vi "TrajectoryCreateExecuteAbsolutePointInFront.vi"(8 "Init":bool, 11 "End Pose ENG":T1={"TRANSLATION"={"X"=0.0, "Y"=0.0}, "ROTATION"={"VALUE"=0.0, "COS"=1.0, "SIN"=0.0}} {"ROTATION"."SIN" format="%13.4f"; "ROTATION"."COS" format="%13.4f"; "ROTATION"."VALUE" format="%13.4f"; "TRANSLATION"."Y" format="%14.3f"; "TRANSLATION"."X" format="%14.3f"}) -> (0 "AtReference":bool, 3 "Chassis Velocity Target":T4 {"vOmega" format="%10.3f"; "vY" format="%10.3f"; "vX" format="%10.3f"})   [LabVIEW 2023]
uses:
  <vilib>/Rock Robotics/WPI/ThirdParty/JAS_Junk/TrajLib/TypeDef/CHASSIS_SPEEDS.ctl
  <vilib>/Rock Robotics/WPI/ThirdParty/JAS_Junk/TrajLib/TypeDef/POSE2D.ctl
  <vilib>/Rock Robotics/WPI/ThirdParty/JAS_Junk/TrajLib/TypeDef/TRANSLATION2D.ctl
  <vilib>/Rock Robotics/WPI/ThirdParty/JAS_Junk/TrajLib/TypeDef/ROTATION2D.ctl
  <vilib>/Rock Robotics/WPI/ThirdParty/JAS_Junk/TrajLib/VI/Util_GetTime_U32.vi
  <vilib>/Rock Robotics/WPI/ThirdParty/JAS_Junk/TrajLib/HolDrvCtrl_New.vi
  <vilib>/Rock Robotics/WPI/ThirdParty/JAS_Junk/TrajLib/HolDrvCtrl_PackPID.vi
  <vilib>/Rock Robotics/WPI/ThirdParty/JAS_Junk/TrajLib/HolDrvCtrl_SetTolerance.vi
  <vilib>/Rock Robotics/WPI/ThirdParty/JAS_Junk/TrajLib/HolDrvCtrl_SetEnabled.vi
  <vilib>/Rock Robotics/WPI/ThirdParty/JAS_Junk/TrajLib/HolDrvCtrl_Calculate_Trajectory.vi
  <vilib>/Rock Robotics/WPI/ThirdParty/JAS_Junk/TrajLib/HolDrvCtrl_AtReference.vi
  <vilib>/Rock Robotics/WPI/ThirdParty/JAS_Junk/TrajLib/ProfiledPIDController_NewPeriod.vi
  <vilib>/Rock Robotics/WPI/ThirdParty/JAS_Junk/TrajLib/ProfiledPIDController_SetIntegratorRange.vi
  <vilib>/Rock Robotics/WPI/ThirdParty/JAS_Junk/TrajLib/ProfiledPIDController_DisableContInput.vi
  <vilib>/Rock Robotics/WPI/ThirdParty/JAS_Junk/TrajLib/ProfiledPIDController_EnableContInput.vi
  <vilib>/Rock Robotics/WPI/ThirdParty/JAS_Junk/TrajLib/TrapProfConstraint_New.vi
  <vilib>/Rock Robotics/WPI/ThirdParty/JAS_Junk/TrajLib/Rotation2d_CreateAngle.vi
  <vilib>/Rock Robotics/WPI/ThirdParty/JAS_Junk/TrajLib/Translation2d_GetXY.vi
  <vilib>/Rock Robotics/WPI/ThirdParty/JAS_Junk/TrajLib/Rotation2d_CreateXY.vi
  <vilib>/Rock Robotics/WPI/ThirdParty/JAS_Junk/TrajLib/Rotation2d_GetRadians.vi
  <vilib>/Rock Robotics/WPI/ThirdParty/JAS_Junk/TrajLib/Conv_Deg_Radians.vi
  <vilib>/Rock Robotics/WPI/ThirdParty/JAS_Junk/TrajLib/PIDController_NewPeriod.vi
  <vilib>/Rock Robotics/WPI/ThirdParty/JAS_Junk/TrajLib/PIDController_SetIntegratorRange.vi
  <vilib>/Rock Robotics/WPI/ThirdParty/JAS_Junk/TrajLib/PIDController_Reset.vi
  <vilib>/Rock Robotics/WPI/ThirdParty/JAS_Junk/TrajLib/HolDrvCtrl_Calculate.vi
  <vilib>/Rock Robotics/WPI/ThirdParty/JAS_Junk/TrajLib/TrapProfState_New.vi
  <vilib>/Rock Robotics/SystemInterfaces/NetworkCommunication/NetComm_UsageReport_report.vi
  <vilib>/Rock Robotics/WPI/ThirdParty/JAS_Junk/TrajLib/PIDController_DisableContinousInput.vi
  <vilib>/Rock Robotics/WPI/ThirdParty/JAS_Junk/TrajLib/PIDController_EnableContinousInput.vi
  <vilib>/Rock Robotics/WPI/ThirdParty/JAS_Junk/TrajLib/Util_CalcDist.vi
  <vilib>/Rock Robotics/WPI/ThirdParty/JAS_Junk/TrajLib/Rotation2d_GetAngleCosSin.vi
  <vilib>/Rock Robotics/WPI/ThirdParty/JAS_Junk/TrajLib/Pose2d_RelativeTo.vi
  <vilib>/Rock Robotics/WPI/ThirdParty/JAS_Junk/TrajLib/Pose2d_getRotation.vi
  <vilib>/Rock Robotics/WPI/ThirdParty/JAS_Junk/TrajLib/Rotation2d_Minus.vi
  <vilib>/Rock Robotics/WPI/ThirdParty/JAS_Junk/TrajLib/ProfiledPIDController_Calculate_Meas_Goal.vi
  <vilib>/Rock Robotics/WPI/ThirdParty/JAS_Junk/TrajLib/PIDController_Calculate_SP_PV.vi
  <vilib>/Rock Robotics/WPI/ThirdParty/JAS_Junk/TrajLib/ProfiledPIDController_Reset_PosOnly.vi
  <vilib>/Rock Robotics/WPI/ThirdParty/JAS_Junk/TrajLib/ChassisSpeeds_FromFieldRelativeSpeeds.vi
  <vilib>/Rock Robotics/WPI/ThirdParty/JAS_Junk/TrajLib/Transform2d_Create_PosePose.vi
  <vilib>/Rock Robotics/WPI/ThirdParty/JAS_Junk/TrajLib/Pose2d_New_TRRO.vi
  <vilib>/Rock Robotics/WPI/ThirdParty/JAS_Junk/TrajLib/Rotation2d_UnaryMinus.vi
  <vilib>/Rock Robotics/WPI/ThirdParty/JAS_Junk/TrajLib/Rotation2d_RotateBy.vi
  <vilib>/Rock Robotics/WPI/ThirdParty/JAS_Junk/TrajLib/ProfiledPIDController_SetGoal_PosOnly.vi
  <vilib>/Rock Robotics/WPI/ThirdParty/JAS_Junk/TrajLib/ProfiledPIDController_Calculate_Meas.vi
  <vilib>/Rock Robotics/WPI/ThirdParty/JAS_Junk/TrajLib/PIDController_SetSetpoint.vi
  <vilib>/Rock Robotics/WPI/ThirdParty/JAS_Junk/TrajLib/PIDController_Calculate_PV.vi
  <vilib>/Rock Robotics/WPI/ThirdParty/JAS_Junk/TrajLib/ProfiledPIDController_Reset.vi
  <vilib>/Rock Robotics/WPI/ThirdParty/JAS_Junk/TrajLib/Rotation2d_GetCos.vi
  <vilib>/Rock Robotics/WPI/ThirdParty/JAS_Junk/TrajLib/Rotation2d_GetSin.vi
  <vilib>/Rock Robotics/WPI/ThirdParty/JAS_Junk/TrajLib/Translation2d_RotateBy.vi
  <vilib>/Rock Robotics/WPI/ThirdParty/JAS_Junk/TrajLib/ProfiledPIDController_SetGoal.vi
  <vilib>/Rock Robotics/WPI/ThirdParty/JAS_Junk/TrajLib/TrapProfile_New.vi
  <vilib>/Rock Robotics/WPI/ThirdParty/JAS_Junk/TrajLib/ProfiledPIDController_GetPeriod.vi
  <vilib>/Rock Robotics/WPI/ThirdParty/JAS_Junk/TrajLib/TrapProfile_Calculate.vi
  <vilib>/Rock Robotics/WPI/ThirdParty/JAS_Junk/TrajLib/ControllerUtil_GetModulusError.vi
  <vilib>/Rock Robotics/WPI/ThirdParty/JAS_Junk/TrajLib/TrapProfile_ShouldFlipAcceleration.vi
  <vilib>/Rock Robotics/WPI/ThirdParty/JAS_Junk/TrajLib/TrapProfile_Direct.vi
  <vilib>/Rock Robotics/WPI/ThirdParty/JAS_Junk/TrajLib/PIDController_GetPeriod.vi
  Vision/VisionGlobal.vi
  TrajectoryGlobals.vi
  <vilib>/Rock Robotics/SystemInterfaces/Utilities/FPGA_UtilitiesRead LocalTime.vi
  <vilib>/Rock Robotics/WPI/ThirdParty/JAS_Junk/TrajLib/VI/Util_GetTime_U64.vi
  <vilib>/Rock Robotics/WPI/ThirdParty/JAS_Junk/TrajLib/Globals/Util_LibraryGlobals.vi
  <vilib>/Rock Robotics/WPI/ThirdParty/JAS_Junk/TrajLib/Trajectory_Library.lvlib
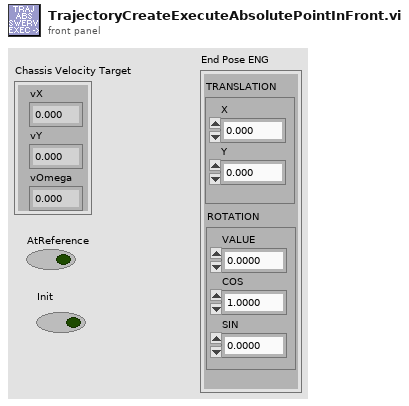
[diagram p1: front panel]
types:
  T1 = typedef "Trajectory_Library.lvlib/POSE2D.ctl" = cluster{"TRANSLATION":T2, "ROTATION":T3}
  T2 = typedef "Trajectory_Library.lvlib/TRANSLATION2D.ctl" = cluster{"X":dbl, "Y":dbl}
  T3 = typedef "Trajectory_Library.lvlib/ROTATION2D.ctl" = cluster{"VALUE":dbl, "COS":dbl, "SIN":dbl}
  T4 = typedef "Trajectory_Library.lvlib/CHASSIS_SPEEDS.ctl" = cluster{"vX":dbl, "vY":dbl, "vOmega":dbl}
  T5 = typedef "Trajectory_Library.lvlib/SWERVE_DRIVE_KINEMATICS.ctl" = cluster{"NumModules":i32, "InverseKinematics":T6, "ForwardKinematics":T6, "Modules":T2[], "PrevCoR":T2, "SavedModuleStates":T7[]}
  T6 = typedef "NI_Matrix.lvlib/RealMatrix.ctl" = dbl[][]
  T7 = typedef "Trajectory_Library.lvlib/SWERVE_DRIVE_MODULE_STATE.ctl" = cluster{"Speed":dbl, "Angle":T3}
  T8 = typedef "Trajectory_Library.lvlib/TRAJECTORY.ctl" = cluster{"TotalTImeSecs":dbl, "States":T9[]}
  T9 = typedef "Trajectory_Library.lvlib/TRAJ_STATE.ctl" = cluster{"TimeSeconds":dbl, "Velocity":dbl, "Acceleration":dbl, "POSE":T1, "Curvature":dbl}
  T10 = typedef "Trajectory_Library.lvlib/PID_TUNING.ctl" = cluster{"Kp":dbl, "Ki":dbl, "Kd":dbl, "MaximumIntegral":dbl, "MinimumIntegral":dbl, "IntegralZone":dbl}
  T11 = typedef "Trajectory_Library.lvlib/PROFILED_PID_CONTROLLER.ctl" = cluster{"Controller":T12, "Goal":T13, "Setpoint":T13, "Constraint":T14}
  T12 = typedef "Trajectory_Library.lvlib/PID_CONTROLLER.ctl" = cluster{"Kp":dbl, "Ki":dbl, "Kd":dbl, "Period":dbl, "Max_Integral":dbl, "Min_Integral":dbl, "Max_Input":dbl, "Min_Input":dbl, "Continuous":bool, "PositionError":dbl, "VelocityError":dbl, "PrevError":dbl, "Total_Integral":dbl, "PositionTolerance":dbl, "VelocityTolerance":dbl, "SetPoint":dbl, "Kf":dbl, "Prev_Deriv":dbl, "Prev_Deriv 2":dbl, "DerivativeFilter":bool, "Min_Output":dbl, "Max_Output":dbl, "Prev_F_P":dbl, "Prev_F_P_2":dbl, "AntiWindupActive":bool, "Measurement":dbl, "IntegralZone":dbl}
  T13 = typedef "Trajectory_Library.lvlib/TRAPEZOID_PROFILE_STATE.ctl" = cluster{"Position":dbl, "Velocity":dbl}
  T14 = typedef "Trajectory_Library.lvlib/TRAPEZOID_PROFILE_CONSTRAINT.ctl" = cluster{"MaxVelocity":dbl, "MaxAcceleration":dbl}
  T15 = typedef "Trajectory_Library.lvlib/HOLONOMIC_PACK_TUNING.ctl" = cluster{"X PID Tuning":T10, "Y PID Tuning":T10, "thetaProfiledPID_CTRL":T11}
  T16 = typedef "Trajectory_Library.lvlib/HOLONOMIC_DRV_CTRL.ctl" = cluster{"poseTolerance":T1, "poseError":T1, "Enabled":bool, "PID_xCtrl":T12, "PID_yCtrl":T12, "PROF_PID_thetaCtrl":T11, "RotationError":T3, "FirstRun":bool}
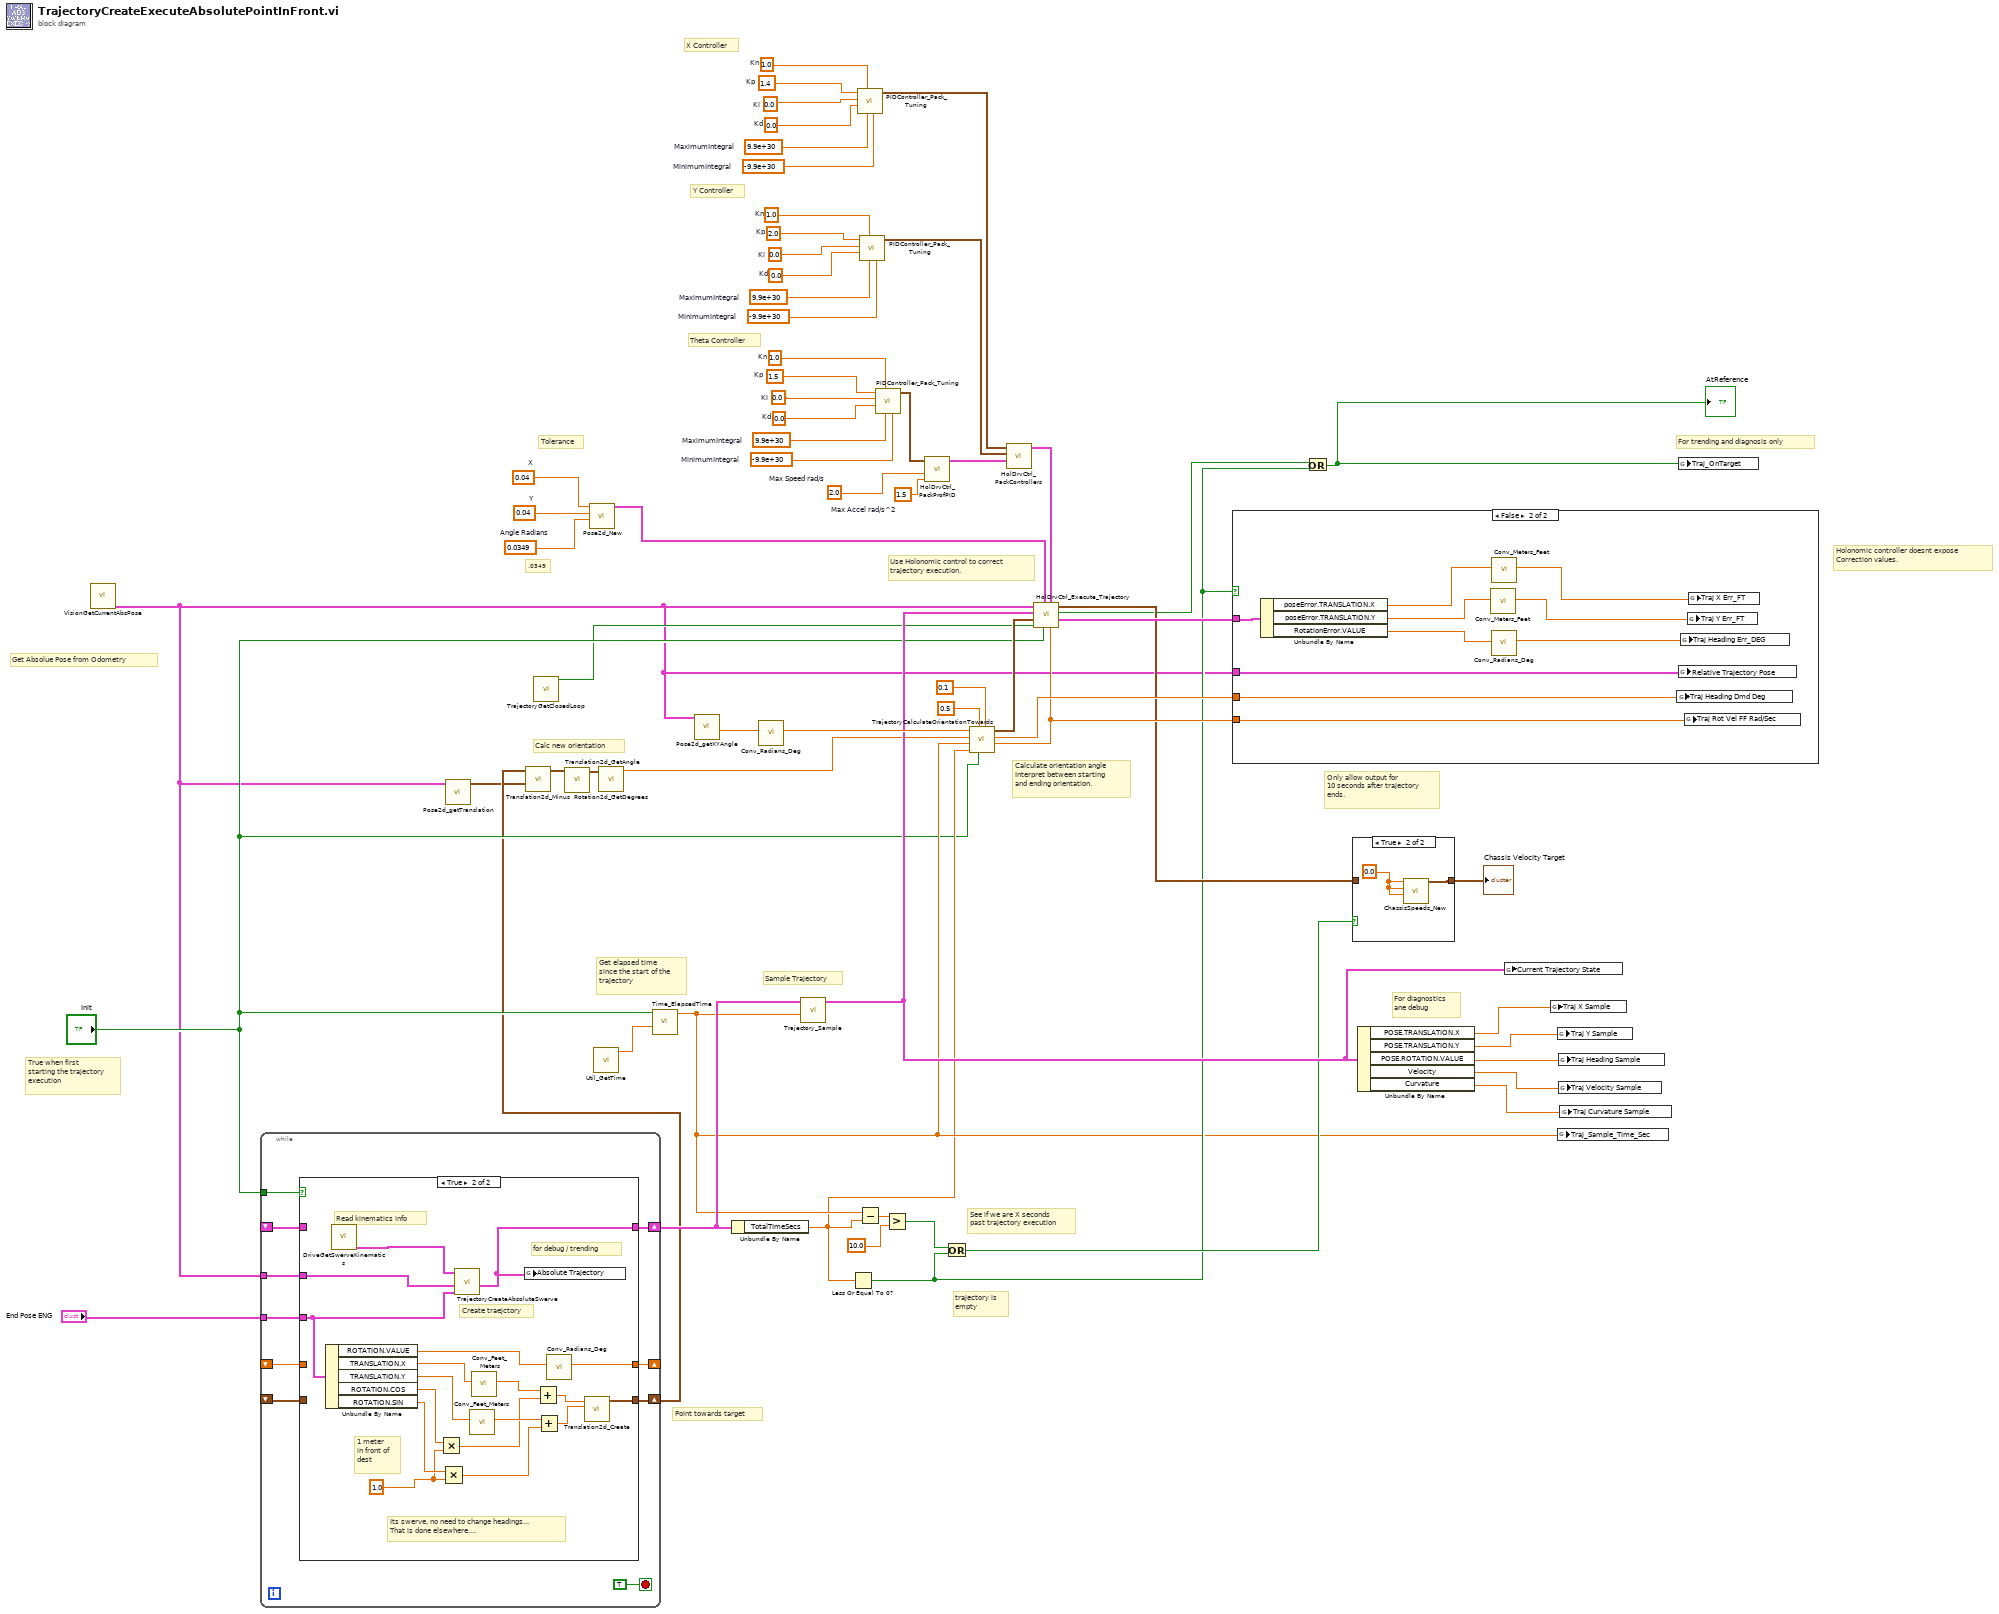
[diagram p0: block diagram]
diagram:
  w11 = 0.04  # X
  w10 = 0.04  # Y
  w12 = 0.0349  # Angle Radians
  w13 = 1.5  # Max Accel rad/s^2
  w14 = 2.0  # Max Speed rad/s
  w36 = 1.0  # Kn
  w39 = 1.5  # Kp
  w48 = 0.0  # Ki
  w49 = 0.0  # Kd
  w50 = 9.9e+30  # MaximumIntegral
  w51 = -9.9e+30  # MinimumIntegral
  w34 = 1.0  # Kn
  w37 = 1.4  # Kp
  w40 = 0.0  # Ki
  w41 = 0.0  # Kd
  w42 = 9.9e+30  # MaximumIntegral
  w43 = -9.9e+30  # MinimumIntegral
  w35 = 1.0  # Kn
  w38 = 2.0  # Kp
  w44 = 0.0  # Ki
  w45 = 0.0  # Kd
  w46 = 9.9e+30  # MaximumIntegral
  w47 = -9.9e+30  # MinimumIntegral
  # "Calc new orientation"
  # "Point towards target"
  # ".0349"
  # "Tolerance"
  # "trajectory is \nempty"
  # "Theta Controller"
  # "Y Controller"
  # "X Controller"
  # "Calculate orientation angle\nInterpret between starting\nand ending orientation."
  # "True when first\nstarting the trajectory\nexecution"
  # "Get elapsed time\nsince the start of the\ntrajectory"
  # "Holonomic controller doesnt expose\nCorrection values."
  # "Use Holonomic control to correct\ntrajectory execution."
  # "For trending and diagnosis only"
  # "For diagnostics\nane debug"
  # "Get Absolue Pose from Odometry"
  # "Sample Trajectory"
  # "See if we are X seconds \npast trajectory execution"
  # "Only allow output for\n10 seconds after trajectory\nends."
  n1 = call "VisionGetCurrentAbsPose.vi"() -> ("Current ABS Pose"=w3:T1)  [unwired: 9 in]
  n2 = while {
    tunnel: "Init" -> [w74]
    tunnel: w3 -> [w73]
    shift-right: [w72] -> w29
    shift-left: _ -> [w71]
    shift-right: [w70] -> _
    shift-left: _ -> [w69]
    tunnel: "End Pose ENG" -> [w68]
    shift-right: [w67] -> w2
    shift-left: _ -> [w66]
    stop <- TRUE stop-if-true
    n3 = case shown="True" w74 {
      tunnel: w73 -> [_ w92]
      tunnel: [w78 w93] -> w72
      tunnel: w71 -> [w78 _]
      tunnel: [w77 w95] -> w70
      tunnel: w69 -> [w77 _]
      tunnel: w68 -> [_ w96]
      tunnel: [w76 w79] -> w67
      tunnel: w66 -> [w76 _]
      frame False {
      }
      frame True {
        w84 = 1.0 ("y")
        # "1 meter\nin front of\ndest"
        # "for debug / trending"
        # "Read kinematics info"
        # "Its swerve, no need to change headings...\nThat is done elsewhere...."
        # "Create traejctory"
        n4 = Unbundle By Name(w96) -> ("ROTATION.VALUE"=w94:dbl, "TRANSLATION.X"=w90:dbl, "TRANSLATION.Y"=w89:dbl, "ROTATION.COS"=w86:dbl, "ROTATION.SIN"=w85:dbl)
        n5 = call "DriveGetSwerveKinematics.vi"() -> ("SWERVE_DRIVE_KINEMATICS"=w91:T5)  [unwired: 11 in]
        n6 = Multiply(x=w86, y=w84) -> (x*y=w83:dbl)
        n7 = Multiply(x=w85, y=w84) -> (x*y=w82:dbl)
        n8 = call "TrajectoryCreateAbsoluteSwerve.vi"("End Pose  ENG"=w96, "Current Pose SI"=w92, "SWERVE_DRIVE_KINEMATICS"=w91) -> ("Absolute Trajectory"=w93:T8)  [unwired: 6 in, 2 out]
        n9 = call <vilib>:"Conv_Feet_Meters.vi"("Feet"=w89) -> ("Meters"=w87:dbl)  [unwired: 10 in]
        n10 = call <vilib>:"Conv_Feet_Meters.vi"("Feet"=w90) -> ("Meters"=w88:dbl)  [unwired: 10 in]
        n11 = global write "TrajectoryGlobals.vi" "Absolute Trajectory"(w93) -> ()
        n12 = Add(x=w88, y=w83) -> (x+y=w81:dbl)
        n13 = Add(x=w87, y=w82) -> (x+y=w80:dbl)
        n14 = call <vilib>:"Conv_Radians_Deg.vi"("Radians"=w94) -> ("Degrees"=w95:dbl)  [unwired: 10 in]
        n15 = call <vilib>:"Translation2d_Create.vi"("Y"=w80, "X"=w81) -> ("TRANSLATION"=w79:T2)  [unwired: 9 in]
      }
    }
  }
  n16 = call <vilib>:"Pose2d_getTranslation.vi"("in POSE"=w3) -> ("outTRANSLATION"=w1:T2)  [unwired: 10 in]
  n17 = call <vilib>:"Translation2d_Minus.vi"("other Translation"=w1, "In Translation"=w2) -> ("Out Translation"=w6:T2)  [unwired: 9 in]
  n18 = call "TrajectoryGetClosedLoop.vi"() -> ("AUTO_CLOSED_LOOP"=w15:bool)  [unwired: 11 in]
  n19 = call <vilib>:"Translation2d_GetAngle.vi"("In Translation"=w6) -> ("Angle_Rotation2d"=w5:T3)  [unwired: 10 in]
  n20 = call <vilib>:"Pose2d_New.vi"("Heading"=w12, "Y"=w10, "X"=w11) -> ("out POSe"=w9:T1)  [unwired: 8 in]
  n21 = call <vilib>:"Util_GetTime.vi"() -> ("FPGA_Time_Seconds"=w62:dbl)  [unwired: 9 in, 2 out]
  n22 = call <vilib>:"Rotation2d_GetDegrees.vi"("in ROTATION"=w5) -> ("AngleDegrees"=w4:dbl)  [unwired: 10 in]
  n23 = call <vilib>:"Time_ElapsedTime.vi"("PassthroughTime_SEC"=w62, "Reset"="Init") -> ("Elapsed Time Sec"=w18:dbl)  [unwired: 9 in]
  n24 = call <vilib>:"Pose2d_getXYAngle.vi"("in POSE"=w3) -> ("Angle"=w28:dbl)  [unwired: 8 in, 2 out]
  n25 = Unbundle By Name(w29) -> ("TotalTImeSecs"=w17:dbl)
  n26 = call <vilib>:"Conv_Radians_Deg.vi"("Radians"=w28) -> ("Degrees"=w27:dbl)  [unwired: 10 in]
  n27 = call <vilib>:"Trajectory_Sample.vi"("Time"=w18, "InputTRAJECTORY"=w29) -> ("OutputTRAJ_STATE"=w26:T9)  [unwired: 9 in]
  n28 = Less Or Equal To 0?(x=w17) -> (x <= 0?=w19:bool)
  n29 = call <vilib>:"PIDController_Pack_Tuning.vi"("MinimumIntegral"=w43, "MaximumIntegral"=w42, "Kn"=w34, "Kd"=w41, "Ki"=w40, "Kp"=w37) -> ("PID Tuning"=w52:T10)  [unwired: 5 in]
  n30 = Subtract(x=w18, y=w17) -> (x-y=w65:dbl)
  n31 = call <vilib>:"PIDController_Pack_Tuning.vi"("MinimumIntegral"=w47, "MaximumIntegral"=w46, "Kn"=w35, "Kd"=w45, "Ki"=w44, "Kp"=w38) -> ("PID Tuning"=w53:T10)  [unwired: 5 in]
  n32 = call <vilib>:"PIDController_Pack_Tuning.vi"("MinimumIntegral"=w51, "MaximumIntegral"=w50, "Kn"=w36, "Kd"=w49, "Ki"=w48, "Kp"=w39) -> ("PID Tuning"=w33:T10)  [unwired: 5 in]
  n33 = Greater?(x=w65, y=10.0) -> (0:w23:bool)
  n34 = call <vilib>:"HolDrvCtrl_PackProfPID.vi"("Max Accel"=w13, "Max Speed"=w14, "Theta PID Tuning"=w33) -> ("Theta PID CONTROLLER"=w54:T11)  [unwired: 8 in]
  n35 = Or(x=w23, y=w19) -> (x .or. y?=w22:bool)
  n36 = call "TrajectoryCalculateOrientationTowards.vi"("Starting Fraction"=0.1, "Init"="Init", "Completion Fraction"=0.5, "Total Trajectory Time Sec"=w17, "Elapsed Traj Time Sec"=w18, "Current Orientation Demand DEG"=w4, "Starting Orientation  DEG"=w27) -> ("Rotational Velocity Rad Per Sec"=w30:dbl, "Orientation Demand Deg"=w56:dbl, "Orientation Demand"=w32:T3)  [unwired: 2 in]
  n37 = call <vilib>:"HolDrvCtrl_PackControllers.vi"("thetaProfiledPID_CTRL"=w54, "Y PID Tuning"=w53, "X PID Tuning"=w52) -> ("HOLONOMIC_CTRL_PACK_TUNING"=w55:T15)  [unwired: 8 in]
  n38 = call <vilib>:"HolDrvCtrl_Execute_Trajectory.vi"("Rotational Velocity Feedforward \nRad/Sec"=w30, "HOLONOMIC_CTRL_PACK_TUNING"=w55, "Reset"="Init", "Tolerance"=w9, "Enable"=w15, "angleRef"=w32, "desiredTrajState"=w26, "currentPose"=w3) -> ("outHOLONOMIC_DRV_CTRL"=w31:T16, "AtReference"=w21:bool, "calcChassisSpeed"=w24:T4)  [unwired: 1 in]
  n39 = case shown="False" w19 {
    tunnel: w56 -> [_ w106]
    tunnel: w31 -> [_ w100]
    tunnel: w30 -> [_ w99]
    tunnel: w3 -> [_ w97]
    frame True {
    }
    frame False {
      n40 = Unbundle By Name(w100) -> ("poseError.TRANSLATION.X"=w104:dbl, "poseError.TRANSLATION.Y"=w103:dbl, "RotationError.VALUE"=w98:dbl)
      n41 = call <vilib>:"Conv_Meters_Feet.vi"("Meters"=w103) -> ("Feet"=w102:dbl)  [unwired: 10 in]
      n42 = call <vilib>:"Conv_Radians_Deg.vi"("Radians"=w98) -> ("Degrees"=w105:dbl)  [unwired: 10 in]
      n43 = call <vilib>:"Conv_Meters_Feet.vi"("Meters"=w104) -> ("Feet"=w101:dbl)  [unwired: 10 in]
      n44 = global write "TrajectoryGlobals.vi" "Traj Heading Dmd Deg"(w106) -> ()
      n45 = global write "TrajectoryGlobals.vi" "Relative Trajectory Pose"(w97) -> ()
      n46 = global write "TrajectoryGlobals.vi" "Traj Heading Err_DEG"(w105) -> ()
      n47 = global write "TrajectoryGlobals.vi" "Traj Rot Vel FF Rad/Sec"(w99) -> ()
      n48 = global write "TrajectoryGlobals.vi" "Traj Y Err_FT"(w102) -> ()
      n49 = global write "TrajectoryGlobals.vi" "Traj X Err_FT"(w101) -> ()
    }
  }
  n50 = Or(x=w21, y=w19) -> (x .or. y?=w20:bool)
  "AtReference" <- w20
  n51 = case shown="True" w22 {
    tunnel: w24 -> [w107 _]
    tunnel: [w107 w108] -> w63
    frame False {
    }
    frame True {
      w109 = 0.0 ("vX")
      n52 = call <vilib>:"ChassisSpeeds_New.vi"("vAngular"=w109, "vY"=w109, "vX"=w109) -> ("CHASSIS"=w108:T4)  [unwired: 8 in]
    }
  }
  "Chassis Velocity Target" <- w63
  n53 = Unbundle By Name(w26) -> ("POSE.TRANSLATION.X"=w61:dbl, "POSE.TRANSLATION.Y"=w60:dbl, "POSE.ROTATION.VALUE"=w59:dbl, "Velocity"=w58:dbl, "Curvature"=w57:dbl)
  n54 = global write "TrajectoryGlobals.vi" "Current Trajectory State"(w26) -> ()
  n55 = global write "TrajectoryGlobals.vi" "Traj X Sample"(w61) -> ()
  n56 = global write "TrajectoryGlobals.vi" "Traj Y Sample"(w60) -> ()
  n57 = global write "TrajectoryGlobals.vi" "Traj_Sample_Time_Sec"(w18) -> ()
  n58 = global write "TrajectoryGlobals.vi" "Traj Heading Sample"(w59) -> ()
  n59 = global write "TrajectoryGlobals.vi" "Traj Velocity Sample"(w58) -> ()
  n60 = global write "TrajectoryGlobals.vi" "Traj Curvature Sample"(w57) -> ()
  n61 = global write "TrajectoryGlobals.vi" "Traj_OnTarget"(w20) -> ()
